vi "Add file number.vi"(9 "sufix number":u32, 11 "file path":path) -> (3 "incremented file path":path)   [LabVIEW 2015, in "VIPM2.lvlib"]
doc: "Concatenates a suffix inside the file name."
uses:
  VIPM2.lvlib
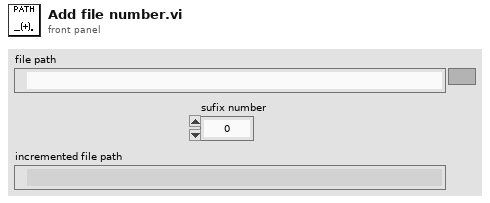
[diagram p1: front panel]
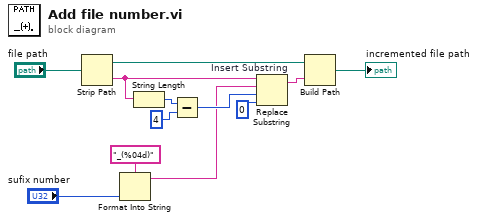
[diagram p0: block diagram]
diagram:
  n1 = Strip Path(path="file path") -> (stripped path=w6:path, name=w10:string)
  n2 = Format Into String "Format Into String"(format string="_(%04d)", "sufix number") -> (resulting string=w1:string)  [unwired: 2 in, 1 out]
  n3 = String Length(string=w10) -> (length=w12:i32)
  n4 = Subtract(x=w12, y=4) -> (x-y=w9:i32)
  n5 = Replace Substring "Insert Substring"(2:0 ("length (len. of substring)"), 3:w9, 4:w1, 5:w10) -> (1:w7:string)  [unwired: 1 out]
  n6 = Build Path(base path=w6, name or relative path=w7) -> (appended path=→"incremented file path":path)
